vi "CTRE_Phoenix_CANifier_SetParameter.vi"(0 "PigeonIMUDevRef":T1={"DeviceStatus"={"status"=FALSE, "code"=0, "source"=""}, "Device Number"=0, "Type"=352321536, "Device ID"=0, "Handle"=0, "UsageFrame"=0, "Library Path"=path ""} {"Type" items=["CAN"=352321536, "TalonSRX"=33554432]}, 5 "Parameter":T3=31 items=["eOnBoot_BrakeMode"=31, "eQuadFilterEn"=91, "eQuadIdxPolarity"=108, "eClearPositionOnIdx"=100, "eMotionProfileHasUnderrunErr"=119, "eClearPosOnLimitF"=144, "eClearPosOnLimitR"=145, "eStatusFramePeriod"=300, "eOpenLoopRamp"=301, "eClosedLoopRamp"=302, "eNeutralDeadband"=303, "ePeakPosOutput"=305, "eNominalPosOutput"=306, "ePeakNegOutput"=307, "eNominalNegOutput"=308, "eProfileParamSlot_P"=310, "eProfileParamSlot_I"=311, "eProfileParamSlot_D"=312, "eProfileParamSlot_F"=313, "eProfileParamSlot_IZone"=314, "eProfileParamSlot_AllowableErr"=315, "eProfileParamSlot_MaxIAccum"=316, "eClearPositionOnLimitF"=320, "eClearPositionOnLimitR"=321, "eClearPositionOnQuadIdx"=322, "eSampleVelocityPeriod"=325, "eSampleVelocityWindow"=326, "eFeedbackSensorType"=330, "eSelectedSensorPosition"=331, "eFeedbackNotContinuous"=332, "eRemoteSensorSource"=333, "eRemoteSensorDeviceID"=334, "eSensorTerm"=335, "eRemoteSensorClosedLoopDisableNeutralOnLOS"=336, "eForwardSoftLimitThreshold"=340, "eReverseSoftLimitThreshold"=341, "eForwardSoftLimitEnable"=342, "eReverseSoftLimitEnable"=343, "eNominalBatteryVoltage"=350, "eBatterVoltageFilterSize"=351, "eContinuousCurrentLimitAmps"=360, "eContinuousCurrentLimitMs"=361, "ePeakCurrentLimitAmps"=362, "eClosedLoopIAccum"=370, "eCustomParam"=380, "eStickyFaults"=390, "eAnalogPosition"=400, "eQuadraturePosition"=401, "ePulseWidthPosition"=402, "eMotMag_Accel"=410, "eMotMag_VelCruise"=411, "eLimitSwitchSource"=421, "eLimitSwitchNormClosedAndDis"=422, "eLimitSwitchDisabledNeutralOnLOS"=423, "eLimitSwitchRemoteDevID"=424], 7 "value":dbl, 9 "subValue":u8, 11 "error in":errorcluster, 12 "ordinal":i32, 13 "timeoutMs":i32) -> (4 "PigeonIMUDevRef":T1={"DeviceStatus"={"status"=FALSE, "code"=0, "source"=""}, "Device Number"=0, "Type"=352321536, "Device ID"=0, "Handle"=0, "UsageFrame"=0, "Library Path"=path ""} {"Type" items=["CAN"=352321536, "TalonSRX"=33554432]}, 15 "error out":errorcluster)   [LabVIEW 2017]
doc: "Sets the parameter value."
uses:
  Controls/CTRE_Phoenix_Params.ctl
  CTRE_PigeonIMU_DeviceRef.ctl
  CTRE_PigeonIMU_ConnectionType.ctl
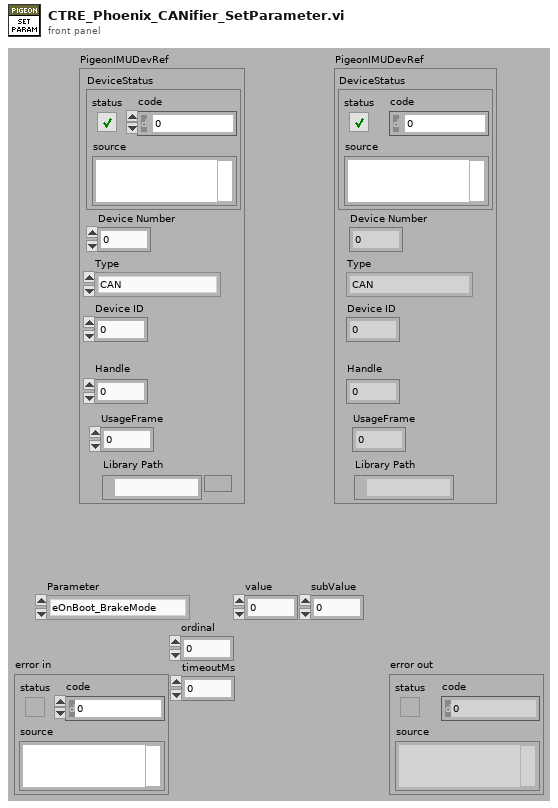
[diagram p1: front panel]
types:
  T1 = typedef "CTRE_PigeonIMU_DeviceRef.ctl" = cluster{"DeviceStatus":errorcluster, "Device Number":u8, "Type":T2, "Device ID":u32, "Handle":u64, "UsageFrame":u32, "Library Path":path}
  T2 = typedef "CTRE_PigeonIMU_ConnectionType.ctl" = u32
  T3 = typedef "CTRE_Phoenix_Params.ctl" = u16
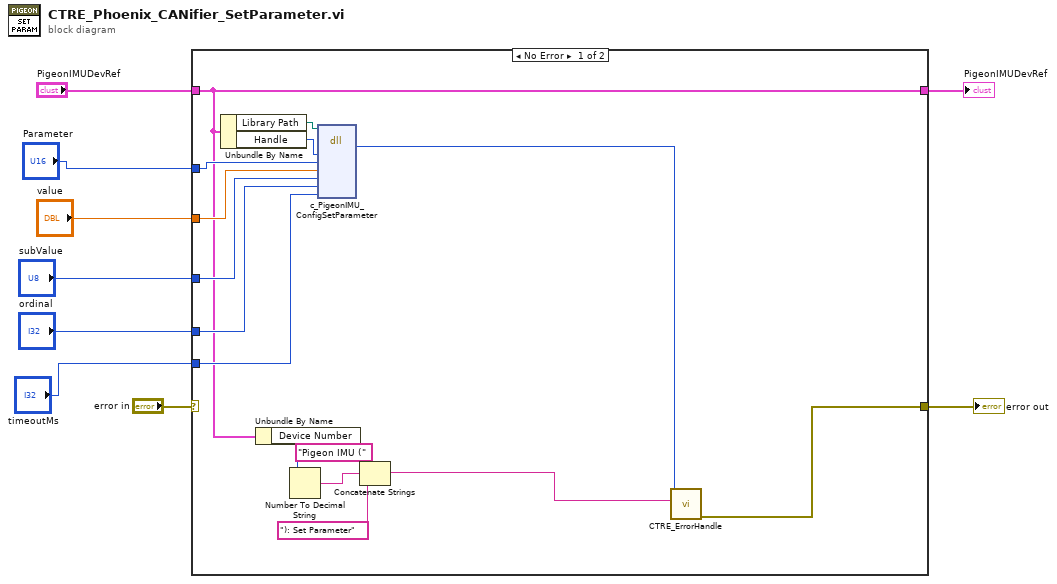
[diagram p0: block diagram]
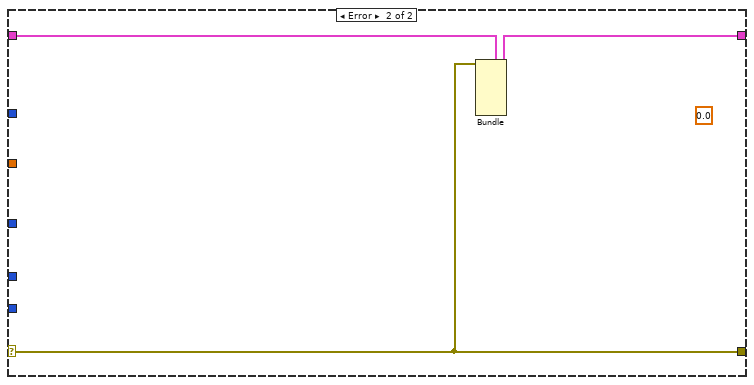
[diagram p2: hidden frame]
diagram:
  n1 = case shown="No Error" "error in" {
    selector: "error in" -> [_ w26]
    tunnel: "PigeonIMUDevRef" -> [w12 w27]
    tunnel: [w24 w26] -> w9
    tunnel: [w12 w25] -> w1
    tunnel: "Parameter" -> [w17 _]
    tunnel: "value" -> [w16 _]
    tunnel: "subValue" -> [w15 _]
    tunnel: "ordinal" -> [w14 _]
    tunnel: "timeoutMs" -> [w13 _]
    frame No Error {
      n2 = Unbundle By Name(w12) -> ("Library Path"=w11:path, "Handle"=w10:u64)
      n3 = Unbundle By Name(w12) -> ("Device Number"=w20:u8)
      n4 = Number To Decimal String(number=w20) -> (decimal integer string=w22:string)  [unwired: 1 in]
      n5 = dll-call lib="?" fn="c_PigeonIMU_ConfigSetParameter"(path in=w11, "handle"=w10, "param"=w17, "value"=w16, "subValue"=w15, "ordinal"=w14, "timeoutMs"=w13) -> ("return type"=w19:i32)  [unwired: 8 in, 2 out]
      n6 = Concatenate Strings("Pigeon IMU (" ("string"), w22, "): Set Parameter" ("string")) -> (w18:string)
      n7 = call "CTRE_ErrorHandle.vi"("origin"=w18, "code"=w19) -> ("error out"=w24:errorcluster)  [unwired: 9 in]
    }
    frame Error {
      (unwired) sgl 0.0 ("value")
      n8 = Bundle(cluster=w27, "DeviceStatus"=w26) -> (w25:T1)  [unwired: 6 in]
    }
  }
  "error out" <- w9
  "PigeonIMUDevRef" <- w1
